vi "P1 Cluster Unwrap.vi"(7 "COM Selector Refs":refnum<vi>[](array[refnum]), 9 "P 1 (App) in":T1) -> (1 "P 1 (App) out":T2, 5 "Initial selection":string[](array[string]))   [LabVIEW 2011]
uses:
  Options Page 1 for display.ctl
  Options Page 1 (App).ctl
panel:
  out "error out":errorcluster
  in  "error in (no error)":errorcluster
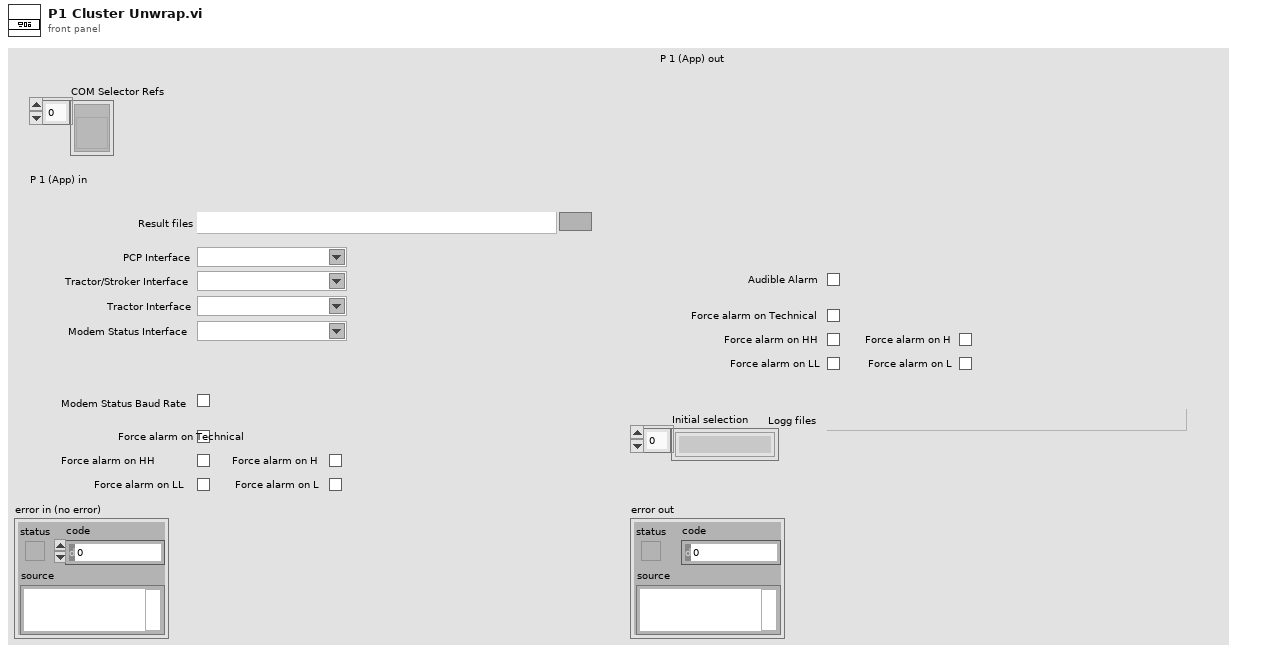
[diagram p1: front panel]
types:
  T1 = typedef "Options Page 1 (App).ctl" = cluster{"Result files":path, "PCP Interface":string, "Tractor/Stroker Interface":string, "Tractor Interface":string, "Modem Status Interface":string, "Audible Alarm":bool, "Force alarm on Technical":bool, "Force alarm on HH":bool, "Force alarm on LL":bool, "Force alarm on H":bool, "Force alarm on L":bool}
  T2 = typedef "Options Page 1 for display.ctl" = cluster{"Logg files":path, "Audible Alarm":bool, "Force alarm on Technical":bool, "Force alarm on HH":bool, "Force alarm on LL":bool, "Force alarm on H":bool, "Force alarm on L":bool}
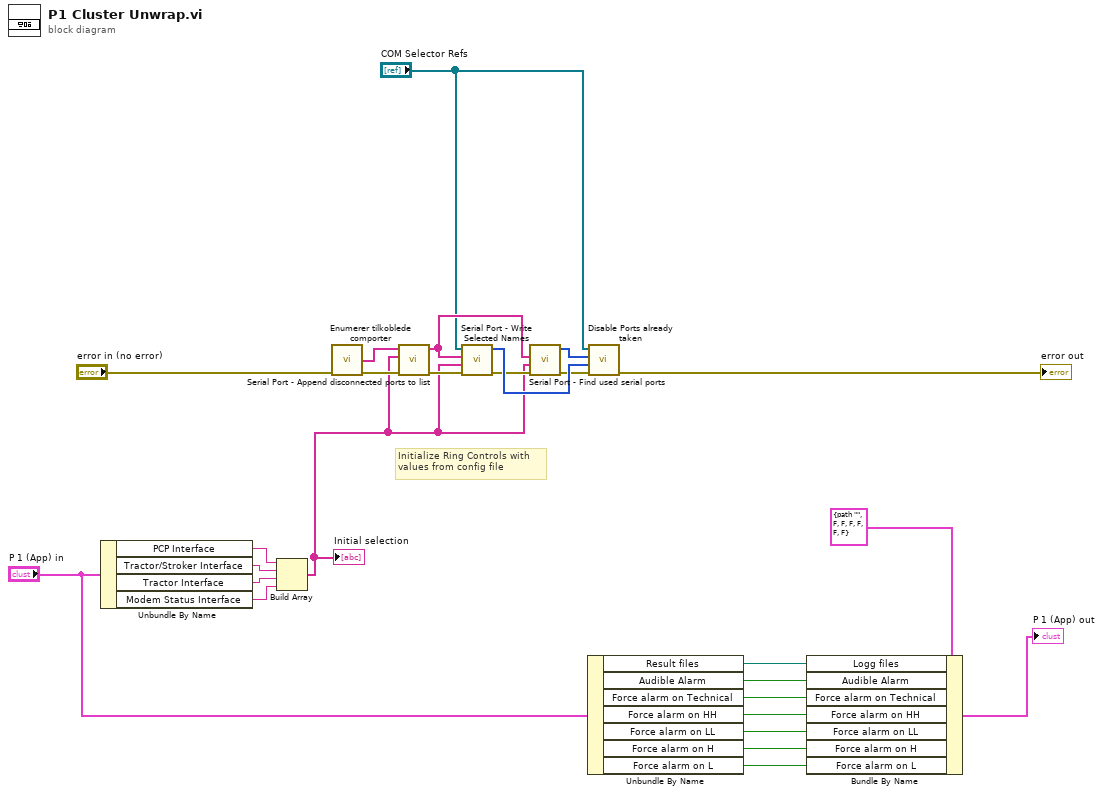
[diagram p0: block diagram]
diagram:
  # "Initialize Ring Controls with \nvalues from config file"
  n1 = Unbundle By Name("P 1 (App) in") -> ("PCP Interface"=w26:string, "Tractor/Stroker Interface"=w25:string, "Tractor Interface"=w24:string, "Modem Status Interface"=w23:string)
  n2 = Build Array(w26, w25, w24, w23) -> (w2:string[])
  "Initial selection" <- w2
  n3 = call "Enumerer tilkoblede comporter.vi"("error in (no error)"="error in (no error)") -> ("Com port w Select string"=w9:string[], "error out"=w10:errorcluster)  [unwired: 11 in, 2 out]
  n4 = call "Serial Port - Append disconnected ports to list.vi"("error in (no error)"=w10, "Selected Values"=w2, "Connected COM Ports in"=w9) -> ("error out"=w7:errorcluster, "COM Ports out"=w8:string[])  [unwired: 7 in]
  n5 = call "Serial Port - Write Selected Names.vi"("error in (no error)"=w7, "Selected Names"=w2, "COM Port List"=w8, "Ctrl Refs in"="COM Selector Refs") -> ("error out"=w6:errorcluster, "Selected Values"=w12:i32[])  [unwired: 6 in]
  n6 = call "Serial Port - Find used serial ports.vi"("error in (no error)"=w6, "Selected Values"=w2, "COM Ports list"=w8) -> ("error out"=w5:errorcluster, "Items to disable"=w11:i32[])  [unwired: 7 in]
  n7 = Unbundle By Name("P 1 (App) in") -> ("Result files"=w19:path, "Audible Alarm"=w18:bool, "Force alarm on Technical"=w17:bool, "Force alarm on HH"=w16:bool, "Force alarm on LL"=w15:bool, "Force alarm on H"=w14:bool, "Force alarm on L"=w13:bool)
  n8 = call "Disable Ports already taken.vi"("error in (no error)"=w5, "Values"=w12, "COM Port numbers taken"=w11, "Ctrl References"="COM Selector Refs") -> ("error out"=→"error out":errorcluster)  [unwired: 7 in]
  n9 = Bundle By Name(cluster=T2 {"Logg files"=path "", "Audible Alarm"=FALSE, "Force alarm on Technical"=FALSE, "Force alarm on HH"=FALSE, "Force alarm on LL"=FALSE, "Force alarm on H"=FALSE, "Force alarm on L"=FALSE} ("P 1 (App)"), "Logg files"=w19, "Audible Alarm"=w18, "Force alarm on Technical"=w17, "Force alarm on HH"=w16, "Force alarm on LL"=w15, "Force alarm on H"=w14, "Force alarm on L"=w13) -> (→"P 1 (App) out":T2)
